vi "MRC IMU Get Acceleration.vi"(8 "error in (no error)":errorcluster) -> (0 "error out":errorcluster, 3 "acceleration":T1)   [LabVIEW 2026, in "MrcLib.lvlib"]
doc: "MRC_Status MRC_CALLCONV MRC_IMU_GetAcceleration(struct MRC_Acceleration3d* acceleration);"
uses:
  MrcLib.lvlib
  Types/MRC 3D Acceleration.ctl
  MrcLib.dll
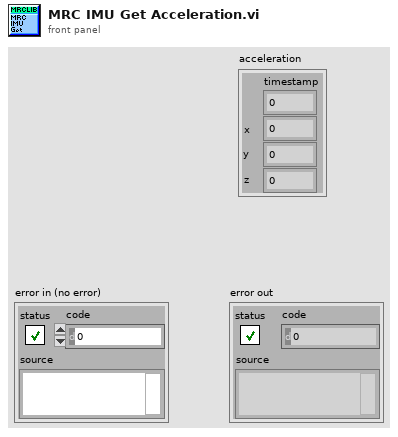
[diagram p1: front panel]
types:
  T1 = typedef "MrcLib.lvlib/MRC 3D Acceleration.ctl" = cluster{"timestamp":i64, "x":dbl, "y":dbl, "z":dbl}
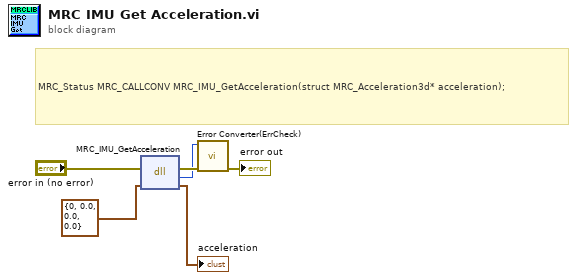
[diagram p0: block diagram]
diagram:
  # "MRC_Status MRC_CALLCONV MRC_IMU_GetAcceleration(struct MRC_Acceleration3d* acceleration);"
  n1 = dll-call lib="MrcLib.*" fn="MRC_IMU_GetAcceleration"(error in="error in (no error)", "acceleration"=T1 {"timestamp"=0, "x"=0.0, "y"=0.0, "z"=0.0} ("accel")) -> (error out=w3:errorcluster, w1:i32, "acceleration"=→"acceleration":T1)  [unwired: 2 in, 1 out]
  n2 = call "Error Converter(ErrCheck).vi"("error in (no error)"=w3, "status"=w1) -> ("error out"=→"error out":errorcluster)  [unwired: 9 in]
